vi "test_SICKTIM571.vi"() -> ()   [LabVIEW 2019]
panel:
  out "Sensor data Graph":cluster{sgl[], sgl[]}(graph)
  out "TIM_XY_DATA":cluster{"X":sgl, "Y":sgl}[](array[cluster])
  in  "stop":bool
  out "data out":string
  in  "TIM571 IP":string="192.168.0.2"
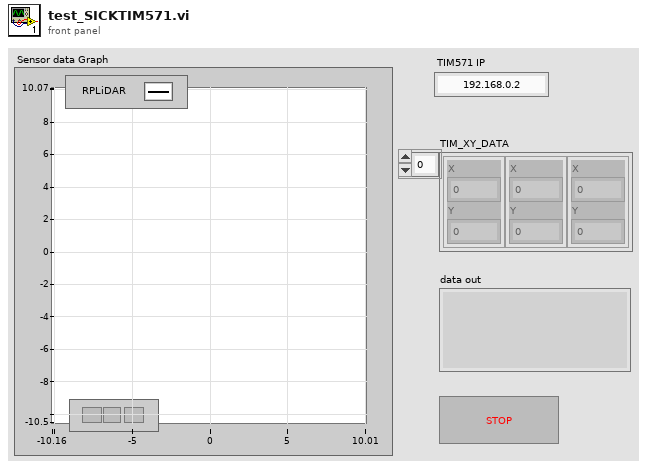
[diagram p1: front panel]
types:
  T1 = enum16{"Standard", "Buffered", "CRLF", "Immediate"}
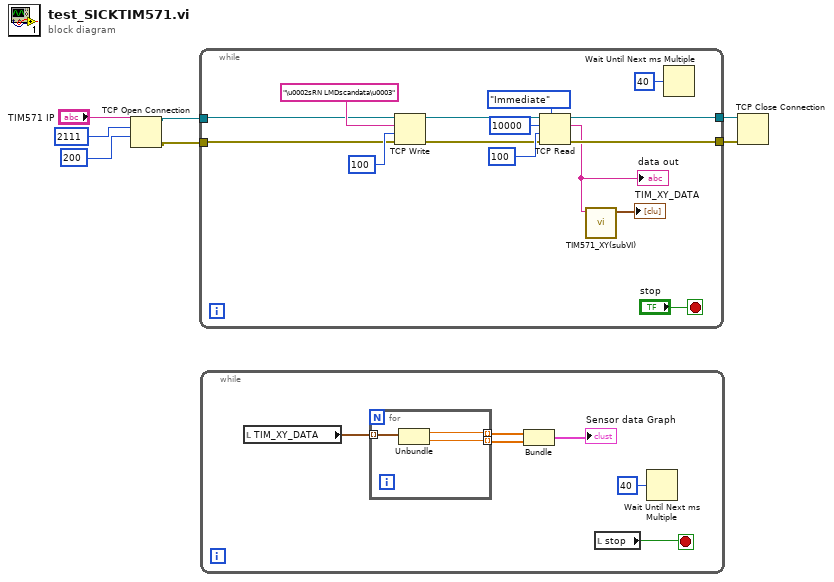
[diagram p0: block diagram]
diagram:
  n1 = TCP Open Connection(address="TIM571 IP", remote port or service name=u16 2111 ("원격 포트 또는 서비스 이름"), timeout ms (60000)=u16 200 ("원격 포트 또는 서비스 이름")) -> (connection ID=w4:refnum<k5>, error out=w3:errorcluster)  [unwired: 2 in]
  n2 = while {
    tunnel: w4 -> [w20]
    tunnel: w3 -> [w19]
    tunnel: [w13] -> w2
    tunnel: [w12] -> w1
    stop <- "stop" stop-if-true
    n3 = TCP Write(connection ID=w20, data in="\u0002sRN LMDscandata\u0003", error in (no error)=w19, 9:100 ("타임아웃 ms (25000)")) -> (connection ID out=w15:refnum<k5>, error out=w14:errorcluster)  [unwired: 1 out]
    n4 = TCP Read(connection ID=w15, bytes to read=10000, error in (no error)=w14, 7:T1."Immediate" ("mode (standard)"), 9:100 ("타임아웃 ms (25000)")) -> (connection ID out=w13:refnum<k5>, data out=w9:string, error out=w12:errorcluster)
    "data out" <- w9
    n5 = call "TIM571_XY(subVI).vi"("input data"=w9) -> ("TIM_XY_DATA"=→"TIM_XY_DATA":cluster{"X":sgl, "Y":sgl}[])  [unwired: 9 in, 1 out]
    n6 = Wait Until Next ms Multiple(millisecond multiple=u32 40 ("ms 배수")) -> ()  [unwired: 1 out]
  }
  n7 = while {
    stop <- w24 stop-if-true
    n8 = local read "TIM_XY_DATA"() -> (w28:cluster{"X":sgl, "Y":sgl}[])
    n9 = for {
      tunnel: w28 -> [w31] mode=indexing
      tunnel: [w30] -> w27 mode=indexing
      tunnel: [w29] -> w26 mode=indexing
      n10 = Unbundle(w31) -> ("X"=w30:sgl, "Y"=w29:sgl)
    }
    n11 = Bundle(w27, w26) -> (→"Sensor data Graph":cluster{sgl[], sgl[]})  [unwired: 1 in]
    n12 = local read "stop"() -> (w24:bool)
    n13 = Wait Until Next ms Multiple(millisecond multiple=u32 40 ("ms 배수")) -> ()  [unwired: 1 out]
  }
  n14 = TCP Close Connection(connection ID=w2, error in (no error)=w1) -> ()  [unwired: 1 in, 2 out]
